vi "Global - PID.vi"() -> ()   [LabVIEW 2019]
panel:
  out "PID":T1(array[cluster])
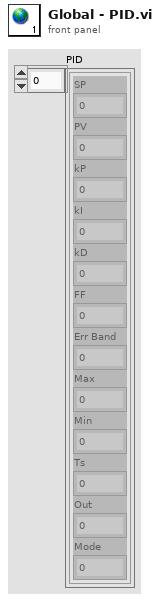
[diagram p1: front panel]
types:
  T1 = cluster{"SP":sgl, "PV":sgl, "kP":sgl, "kI":sgl, "kD":sgl, "FF":sgl, "Err Band":sgl, "Max":i32, "Min":i32, "Ts":u32, "Out":i32, "Mode":u8}[]
diagram:
